vi "SPD.Connection Test.vi"(8 "Error In":errorcluster, 11 "SPD.Stand Ctrl in":T1) -> (0 "Error Out":errorcluster, 1 "HW ok":bool, 2 "HW report":string, 3 "SPD.Stand Ctrl out":T1)   [LabVIEW 2018]
uses:
  typedefs/SPD.Stand Ctrl.ctl
  Instruments/SPD HID Interface/hidSPDLibForLabView/LibVIs/hidSPD Controls/hidSPD Device Session.ctl
  Instruments/KC705 DevBoard/typedefs/DevB.Session.ctl
  Instruments/KeySight 53230A/typedefs/FreqC.Session.ctl
  Instruments/KeySight 8164B/KeySight 8164B LAN InstrLib/typedefs/KeySight 8164B control.ctl
  Instruments/SPD HID Interface/hidSPDLibForLabView/hidSPDLibForLabView.lvlib
  Instruments/KeySight 8164B/KeySight 8164B LAN InstrLib.lvlib
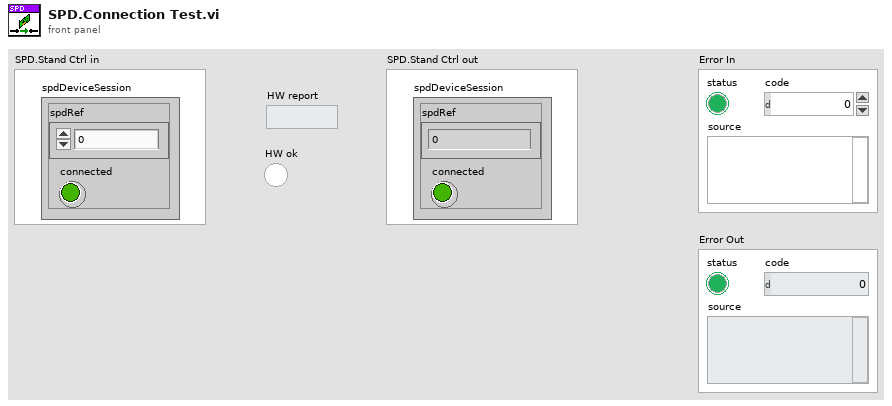
[diagram p1: front panel]
types:
  T1 = typedef "SPD.Stand Ctrl.ctl" = cluster{"spdDeviceSession":T2, "DevBSession":T3, "FreqCSession":T4, "8164BSession":T5}
  T2 = typedef "hidSPDLibForLabView.lvlib/hidSPD Device Session.ctl" = cluster{"spdRef":u64, "connected":bool}
  T3 = typedef "DevB.Session.ctl" = cluster{"DevBRef":refnum<visa-resource-name>, "connected":bool}
  T4 = typedef "FreqC.Session.ctl" = cluster{"FreqCRef":refnum<visa-resource-name>, "timeout":dbl, "connected":bool}
  T5 = typedef "KeySight 8164B LAN InstrLib.lvlib/KeySight 8164B control.ctl" = cluster{"Connection ID":refnum<k5>, "Connected":bool, "Info":string, "Slots Info":string[]}
  T6 = typedef "hidSPDLibForLabView.lvlib/hidSPD HidDevInfo.ctl" = cluster{"name":string, "path":string}
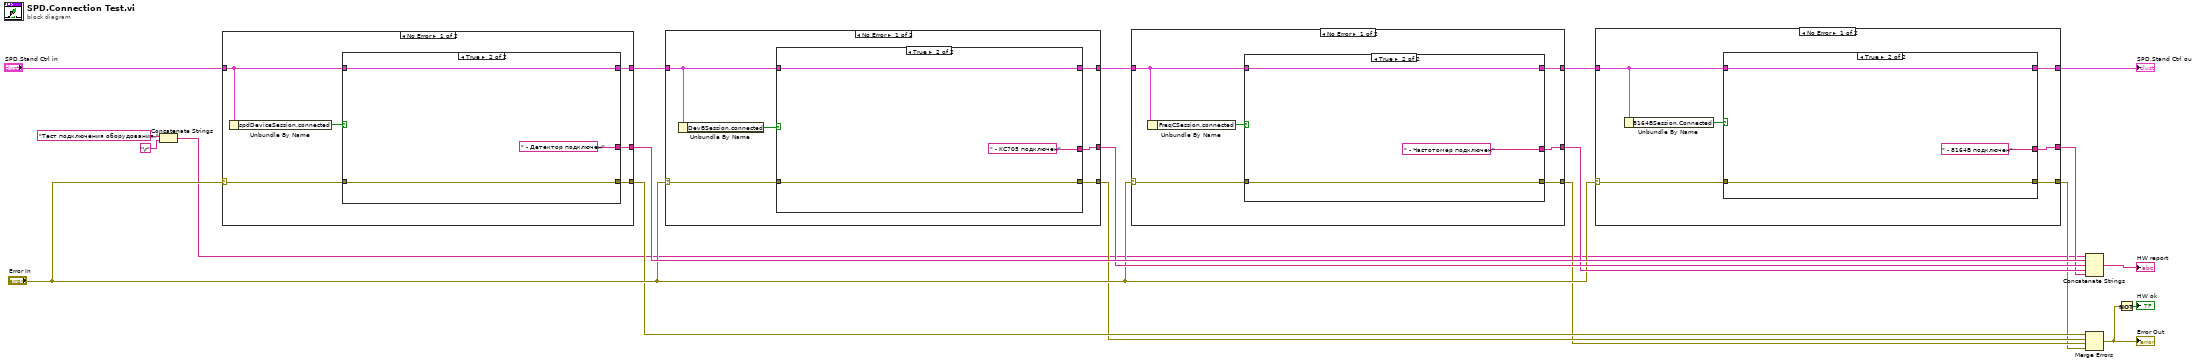
[diagram p0: block diagram]
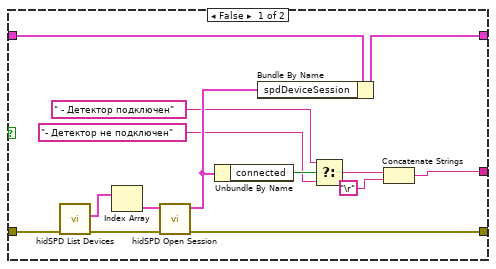
[diagram p2: hidden frame]
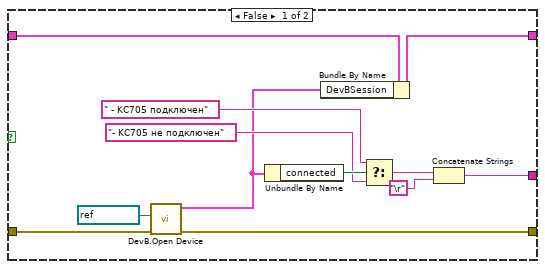
[diagram p4: hidden frame]
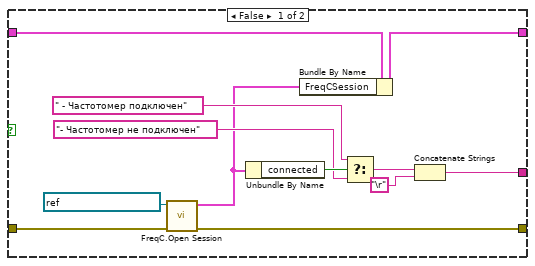
[diagram p6: hidden frame]
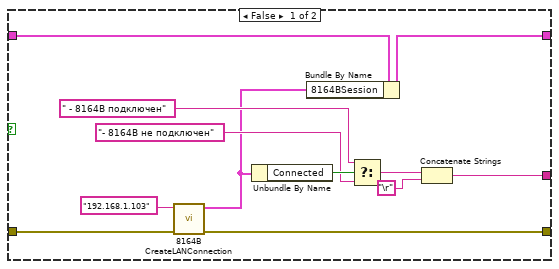
[diagram p8: hidden frame]
diagram:
  n1 = Concatenate Strings("Тест подключения оборудования.", "\r") -> (w1:string)
  n2 = case shown="No Error" "Error In" {
    selector: "Error In" -> [w26 w44]
    tunnel: "SPD.Stand Ctrl in" -> [w22 w45]
    tunnel: [w25 w44] -> w9
    tunnel: [w24 w45] -> w18
    tunnel: [w23 _] -> w19
    frame No Error {
      n3 = Unbundle By Name(w22) -> ("spdDeviceSession.connected"=w21:bool)
      n4 = case shown="True" w21 {
        tunnel: w26 -> [w40 w42]
        tunnel: w22 -> [w36 w43]
        tunnel: [w31 w42] -> w25
        tunnel: [w30 w43] -> w24
        tunnel: [w28 " - Детектор подключен"] -> w23
        frame False {
          n5 = call "hidSPD List Devices.vi"("error in (no error)"=w40) -> ("error out"=w37:errorcluster, "devices list"=w39:T6[])  [unwired: 9 in]
          n6 = Index Array(array=w39) -> (element=w38:T6)  [unwired: 1 in]
          n7 = call "hidSPD Open Session.vi"("error in (no error)"=w37, "HidDevInfo"=w38) -> ("error out"=w31:errorcluster, "spdDevSession out"=w35:T2)  [unwired: 8 in]
          n8 = Unbundle By Name(w35) -> ("connected"=w34:bool)
          n9 = Bundle By Name(cluster=w36, "spdDeviceSession"=w35) -> (w30:T1)
          n10 = Select(t=" - Детектор подключен", s=w34, f="- Детектор не подключен") -> (s? t:f=w29:string)
          n11 = Concatenate Strings(w29, "\r") -> (w28:string)
        }
        frame True {
        }
      }
    }
    frame Error {
    }
  }
  n12 = case shown="No Error" "Error In" {
    selector: "Error In" -> [w49 w67]
    tunnel: w18 -> [w47 w68]
    tunnel: [w48 w67] -> w8
    tunnel: [w51 w68] -> w16
    tunnel: [w50 _] -> w17
    frame No Error {
      n13 = Unbundle By Name(w47) -> ("DevBSession.connected"=w46:bool)
      n14 = case shown="True" w46 {
        tunnel: w47 -> [w63 w66]
        tunnel: [w59 w66] -> w51
        tunnel: [w57 " - KC705 подключен"] -> w50
        tunnel: w49 -> [w55 w65]
        tunnel: [w54 w65] -> w48
        frame False {
          n15 = call "DevB.Open Device.vi"("error in (no error)"=w55, "Port"=refnum<visa-resource-name> "COM3") -> ("error out"=w54:errorcluster, "DevB Session out"=w52:T3)  [unwired: 8 in]
          n16 = Unbundle By Name(w52) -> ("connected"=w62:bool)
          n17 = Bundle By Name(cluster=w63, "DevBSession"=w52) -> (w59:T1)
          n18 = Select(t=" - KC705 подключен", s=w62, f="- KC705 не подключен") -> (s? t:f=w58:string)
          n19 = Concatenate Strings(w58, "\r") -> (w57:string)
        }
        frame True {
        }
      }
    }
    frame Error {
    }
  }
  n20 = case shown="No Error" "Error In" {
    selector: "Error In" -> [w72 w90]
    tunnel: w16 -> [w70 w91]
    tunnel: [w71 w90] -> w7
    tunnel: [w74 w91] -> w14
    tunnel: [w73 _] -> w15
    frame No Error {
      n21 = Unbundle By Name(w70) -> ("FreqCSession.connected"=w69:bool)
      n22 = case shown="True" w69 {
        tunnel: w70 -> [w86 w89]
        tunnel: [w82 w89] -> w74
        tunnel: [w80 " - Частотомер подключен"] -> w73
        tunnel: w72 -> [w77 w88]
        tunnel: [w76 w88] -> w71
        frame False {
          n23 = call "FreqC.Open Session.vi"("error In"=w77, "VISA resource name"=refnum<visa-resource-name> "KeySight_53230A") -> ("error out"=w76:errorcluster, "FreqC Session out"=w75:T4)  [unwired: 8 in]
          n24 = Unbundle By Name(w75) -> ("connected"=w85:bool)
          n25 = Bundle By Name(cluster=w86, "FreqCSession"=w75) -> (w82:T1)
          n26 = Select(t=" - Частотомер подключен", s=w85, f="- Частотомер не подключен") -> (s? t:f=w81:string)
          n27 = Concatenate Strings(w81, "\r") -> (w80:string)
        }
        frame True {
        }
      }
    }
    frame Error {
    }
  }
  n28 = case shown="No Error" "Error In" {
    selector: "Error In" -> [w95 w113]
    tunnel: w14 -> [w93 w114]
    tunnel: [w94 w113] -> w6
    tunnel: [w97 w114] -> w11
    tunnel: [w96 _] -> w13
    frame No Error {
      n29 = Unbundle By Name(w93) -> ("8164BSession.Connected"=w92:bool)
      n30 = case shown="True" w92 {
        tunnel: w93 -> [w109 w112]
        tunnel: [w105 w112] -> w97
        tunnel: [w103 " - 8164B подключен"] -> w96
        tunnel: w95 -> [w100 w111]
        tunnel: [w99 w111] -> w94
        frame False {
          n31 = call "8164B CreateLANConnection.vi"("error in"=w100, "IP address"="192.168.1.103" ("address")) -> ("error out"=w99:errorcluster, "KeySight 8164B control out"=w98:T5)  [unwired: 8 in]
          n32 = Unbundle By Name(w98) -> ("Connected"=w108:bool)
          n33 = Bundle By Name(cluster=w109, "8164BSession"=w98) -> (w105:T1)
          n34 = Select(t=" - 8164B подключен", s=w108, f="- 8164B не подключен") -> (s? t:f=w104:string)
          n35 = Concatenate Strings(w104, "\r") -> (w103:string)
        }
        frame True {
        }
      }
    }
    frame Error {
    }
  }
  "SPD.Stand Ctrl out" <- w11
  n36 = Concatenate Strings(w1, w19, w17, w15, w13) -> (→"HW report":string)
  n37 = Merge Errors(w9, w8, w7, w6) -> (w5:errorcluster)
  "Error Out" <- w5
  n38 = Not(x=w5) -> (.not. x?=→"HW ok":bool)
